vi "GaitEvent.vi"(8 "Right Toe":dbl, 9 "Time(mm)":dbl, 10 "Right Heel":dbl, 11 "bIndIn":bool) -> (0 "bHeelSt":bool, 1 "GaitCylce(%)":dbl, 3 "bIndOut":bool)   [LabVIEW 2017]
uses:
  <vilib>/imath/engines/lvmath2/RunTimeEngine/NodeEndStatement/NIMS_NodeEndStatement_Output.vi
  <instcachedir>/0/NIMS_NodeEndStatement_Output_53EC0D466D134D7ABD903AC30B43404B.lvgen/NIMS_NodeEndStatement_Output_53EC0D466D134D7ABD903AC30B43404B_010.vi
  <vilib>/imath/engines/lvmath2/RunTimeEngine/ErrorHandling/NIMS_Finalize Error.vi
panel:
  in  "ThrL":dbl=2.6
  in  "ThrH":dbl=2.8
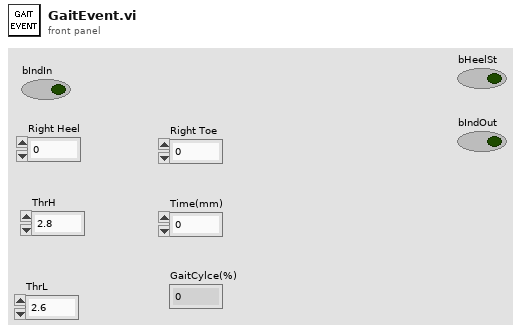
[diagram p1: front panel]
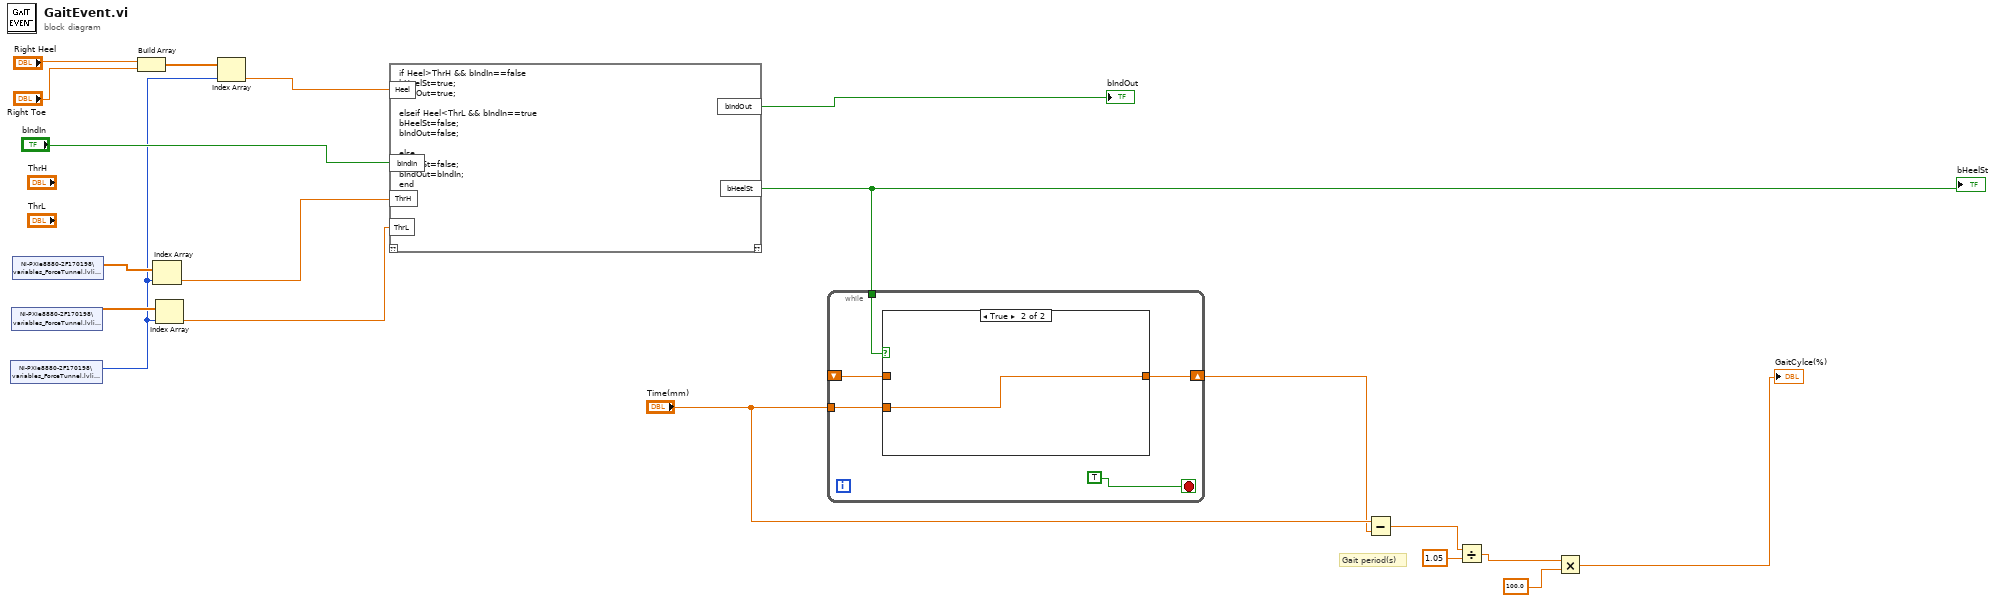
[diagram p0: block diagram]
diagram:
  # "Gait period(s)"
  n1 = shared-variable "NI-PXIe8880-2F170198\\variables_ForceTunnel.lvlib\\iGateEvent"() -> (w3:i16)  [unwired: 1 in, 1 out]
  n2 = shared-variable "NI-PXIe8880-2F170198\\variables_ForceTunnel.lvlib\\GaitThrOff"() -> (w7:dbl[])  [unwired: 1 in, 1 out]
  n3 = shared-variable "NI-PXIe8880-2F170198\\variables_ForceTunnel.lvlib\\GaitThrOn"() -> (w9:dbl[])  [unwired: 1 in, 1 out]
  n4 = Build Array("Right Heel", "Right Toe") -> (w2:dbl[])
  n5 = Index Array(array=w9, index=w3) -> (element=w8:dbl)
  n6 = Index Array(array=w7, index=w3) -> (element=w6:dbl)
  n7 = Index Array(array=w2, index=w3) -> (element=w1:dbl)
  n8 = mathscript code="if Heel>ThrH && bIndIn==false\nbHeelSt=true;\nbIndOut=true;\n\nelseif Heel<ThrL && bIndIn==true\nbHeelSt=false;\nbIndOut=false;\n\nelse\nbHeelSt=false;\nbIndOut=bIndIn;\nend"("Heel"=w1, "bIndIn"="bIndIn", "ThrH"=w8, "ThrL"=w6) -> ("bIndOut"=→"bIndOut":bool, "bHeelSt"=w17:bool)  [unwired: 1 in, 1 out]
  "bHeelSt" <- w17
  n9 = while {
    tunnel: w17 -> [w24]
    shift-right: [w23] -> w11
    shift-left: _ -> [w21]
    tunnel: "Time(mm)" -> [w22]
    stop <- TRUE stop-if-true
    n10 = case shown="True" w24 {
      tunnel: [w25 w26] -> w23
      tunnel: w22 -> [_ w26]
      tunnel: w21 -> [w25 _]
      frame False {
      }
      frame True {
      }
    }
  }
  n11 = Subtract(x="Time(mm)", y=w11) -> (x-y=w15:dbl)
  n12 = Divide(x=w15, y=1.05) -> (x/y=w13:dbl)
  n13 = Multiply(x=w13, y=100.0) -> (x*y=→"GaitCylce(%)":dbl)
